vi "path.vi"() -> ()   [LabVIEW 2020]
panel:
  out "output":string
  in  "input":path
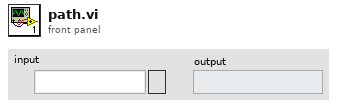
[diagram p1: front panel]
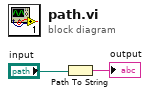
[diagram p0: block diagram]
diagram:
  n1 = Path To String(path="input") -> (string=→"output":string)
